vi "Main.vi"(11 "Module Admin":refnum<class "Delacor_lib_QMH_Module Admin.lvclass">) -> ()   [LabVIEW 2024, in "UI.lvlib"]
doc: "This template is based off of the Queued Message Handler design pattern and the Queued Message Handler project template that ships with LabVIEW.\n\nThe main difference is that the queue is private to this module and communication between modules is performed via Broadcast and Request events.\n\nRequest events are wrapped in public API methods and are handled in the Event Handling Loop (EHL) of this VI. Any module can register for Broadcast events sent by this module. The EHL generates messages based on user interface actions.\n\nThe Message Handling Loop (MHL) processes messages generated by the EHL, or by other messages. The messages are string values, so new messages can be added easily to the Message Cases case structure in the MHL. Each message cluster can also provide an optional value for Message Data, which is a variant that can be converted to whatever message-specific data is required.\n_____\nBased on DQMH Project Template 7.0.1.1316."
uses:
  UI.lvlib
  <vilib>/Delacor/Delacor QMH/Libraries/Message Queue_class/Delacor_lib_QMH_Message Queue.lvclass/Delacor_lib_QMH_Message Queue.ctl
  <vilib>/Delacor/Delacor QMH/Libraries/Module Admin_class/Delacor_lib_QMH_Module Admin.lvclass/Delacor_lib_QMH_Module Admin.ctl
  UI Module Template/Start Module.vi
  UI Module Template/Stop Module.vi
  <vilib>/Delacor/Delacor QMH/Libraries/Message Queue_class/Delacor_lib_QMH_Message Queue.lvclass
  Module Data--cluster.ctl
  <vilib>/Delacor/Delacor QMH/Libraries/Message Queue_class/Delacor_lib_QMH_Enqueue Message (Single).vi
  Stop Argument--cluster.ctl
  <vilib>/Delacor/Delacor QMH/Libraries/Module Admin_class/Delacor_lib_QMH_Module Admin.lvclass
  Start Modules Argument--cluster.ctl
  Modules.ctl
  Display Module Argument--cluster.ctl
  Acquire/Acquire.lvlib
  Explore/Explore.lvlib
  ListViewer/Obtain Broadcast Events for Registration.vi
  ListViewer/ListViewer.lvlib
  DataViewer/Obtain Broadcast Events for Registration.vi
  DataViewer/DataViewer.lvlib
  UI Module Template/UI Module Template.lvlib
panel:
  in  "Buttons":bool[](array[boolean])
  in  "Explore":bool
  in  "Acquisition":bool
  out "Status":string
  out "error out":errorcluster
  out "Status":string
  in  "Simulate MHL Error":bool
  in  "Simulate EHL Error":bool
  # "DQMH UI Demo"
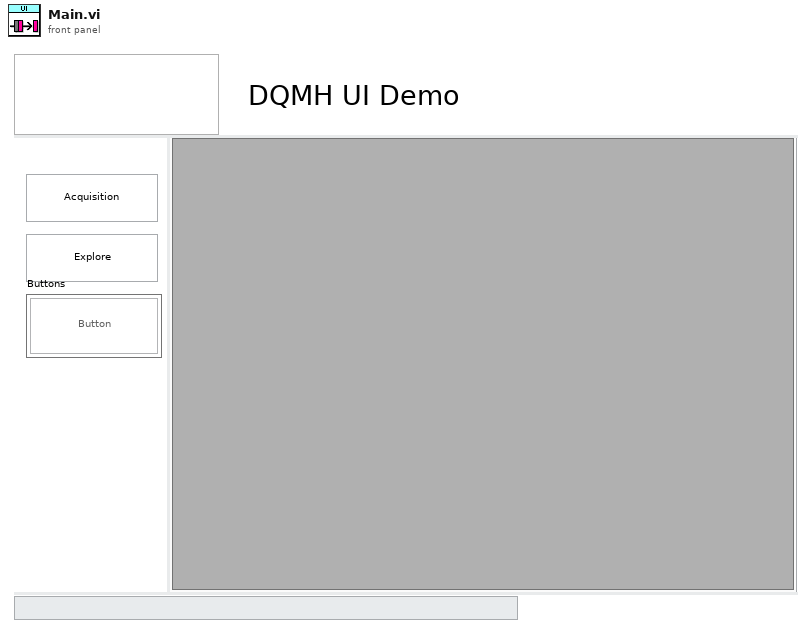
[diagram p1: front panel]
types:
  T1 = typedef "UI.lvlib/Module Data--cluster.ctl" = cluster{"Status":string, "Modules":refnum<vi>[]}
  T2 = typedef "UI.lvlib/Request Events--cluster.ctl" = cluster{"Stop Module":refnum<user-event>, "Show Panel":refnum<user-event>, "Hide Panel":refnum<user-event>, "Get Module Execution Status":refnum<user-event>, "Show Diagram":refnum<user-event>, "Private":cluster{"Start Modules":refnum<user-event>}, "Display Module":refnum<user-event>}
  T3 = typedef "ListViewer.lvlib/Broadcast Events--cluster.ctl" = cluster{"Module Did Init":refnum<user-event>, "Status Updated":refnum<user-event>, "Error Reported":refnum<user-event>, "Module Did Stop":refnum<user-event>, "Update Module Execution Status":refnum<user-event>}
  T4 = typedef "DataViewer.lvlib/Broadcast Events--cluster.ctl" = cluster{"Module Did Init":refnum<user-event>, "Status Updated":refnum<user-event>, "Error Reported":refnum<user-event>, "Module Did Stop":refnum<user-event>, "Update Module Execution Status":refnum<user-event>}
  T5 = enum32{"invalid lock state", "Not Locked", "Locked (No Password)", "Password-protected"}
  T6 = typedef "UI.lvlib/Stop Argument--cluster.ctl" = cluster{"Origin":string, "Exit via Stop Module Req?":bool, "Wait for Module to stop?":bool}
  T7 = typedef "UI.lvlib/Start Modules Argument--cluster.ctl" = cluster{"Boolean":bool}
  T8 = typedef "UI.lvlib/Display Module Argument--cluster.ctl" = cluster{"Modules":T9}
  T9 = typedef "UI.lvlib/Modules.ctl" = enum16{"Explore", "Acquisition"}
  T10 = enum32{"Invalid", "Standard", "Closed", "Hidden", "Minimized", "Maximized"}
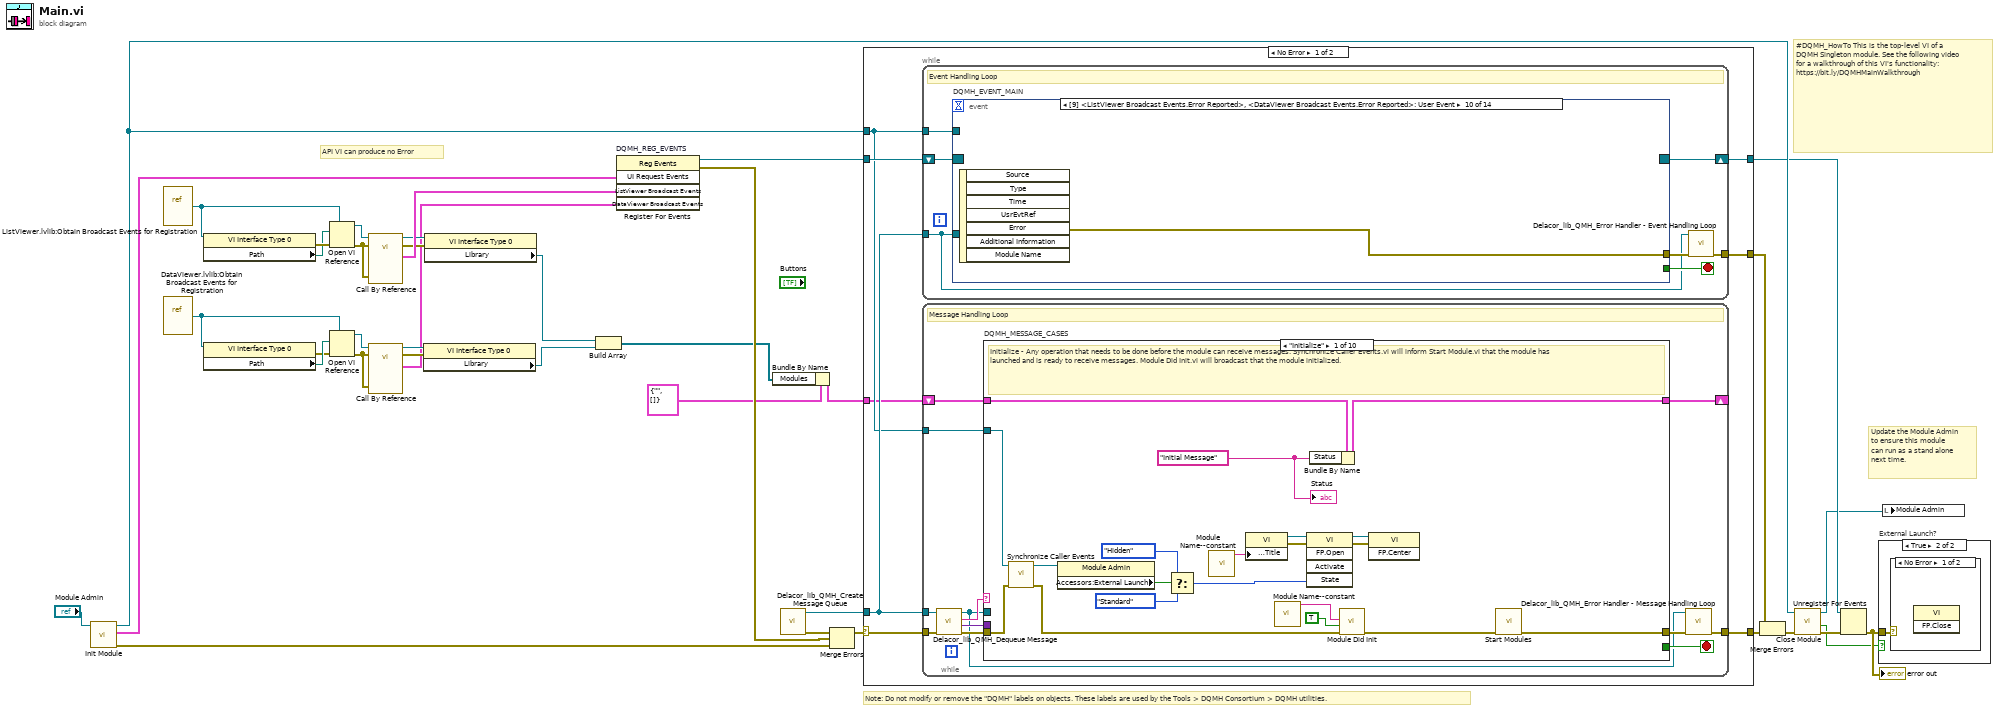
[diagram p0: block diagram]
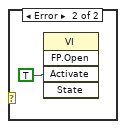
[diagram p3: hidden frame]
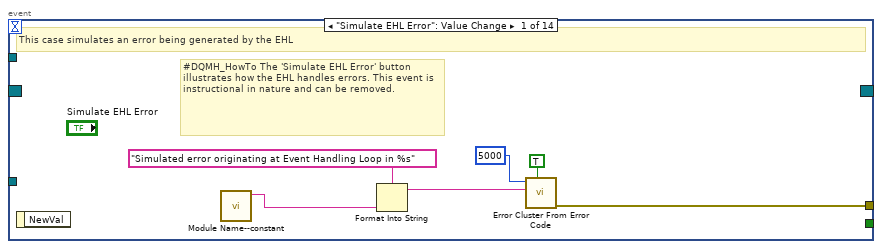
[diagram p4: hidden frame]
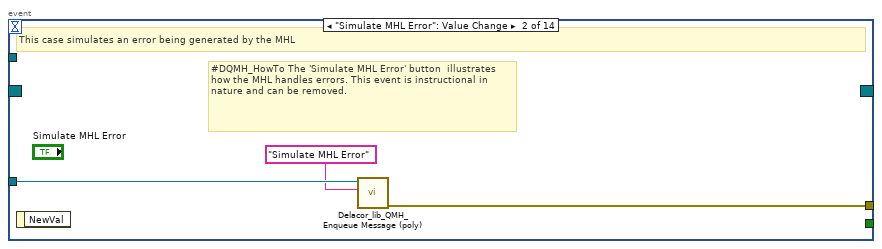
[diagram p5: hidden frame]
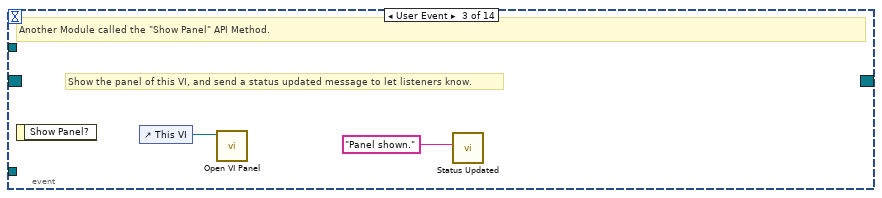
[diagram p6: hidden frame]
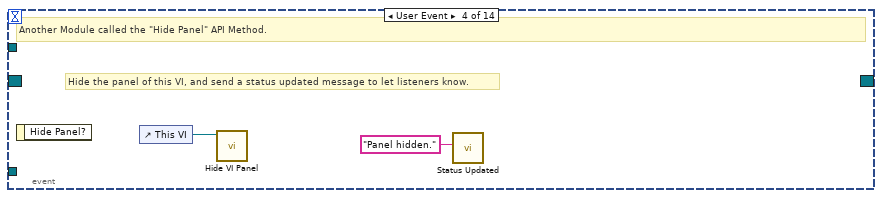
[diagram p7: hidden frame]
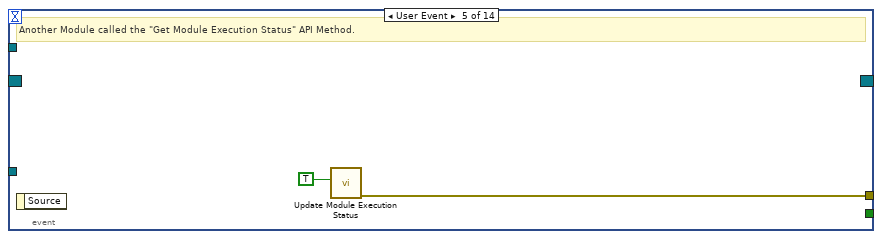
[diagram p8: hidden frame]
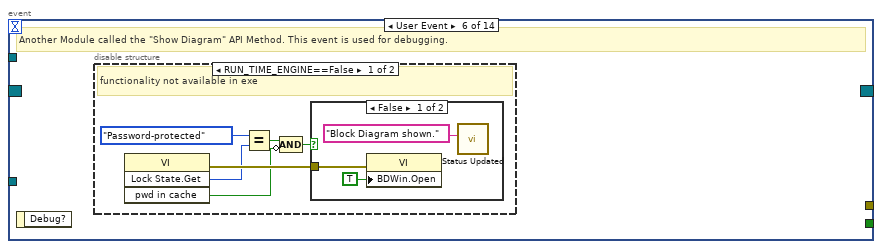
[diagram p9: hidden frame]
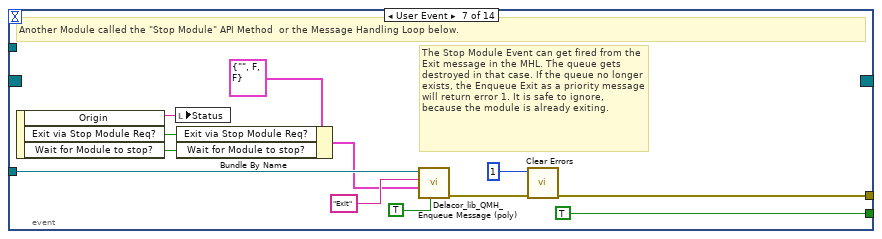
[diagram p12: hidden frame]
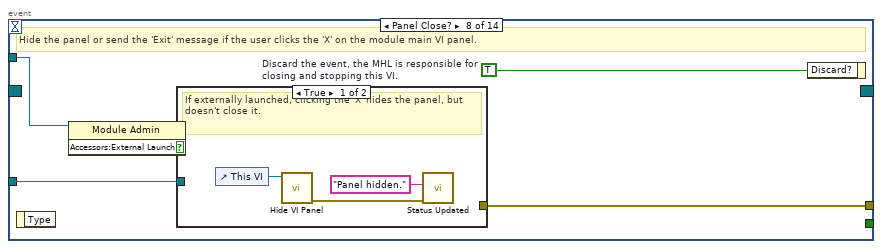
[diagram p13: hidden frame]
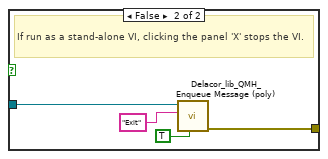
[diagram p14: hidden frame]
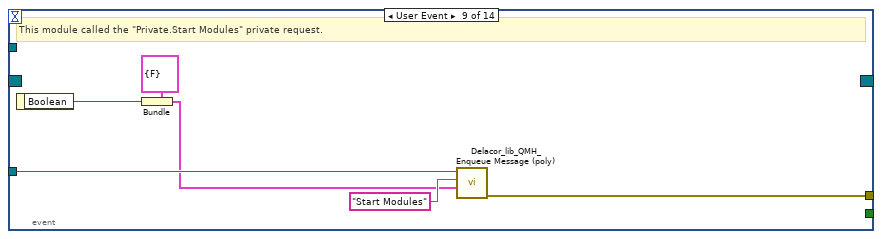
[diagram p15: hidden frame]
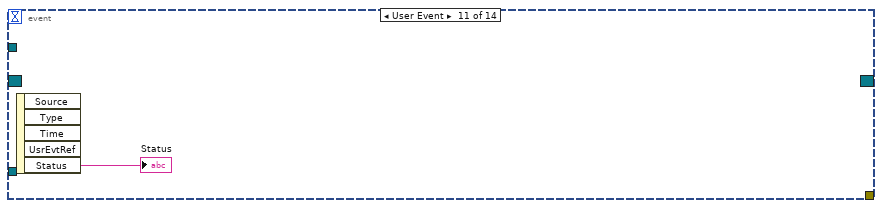
[diagram p16: hidden frame]
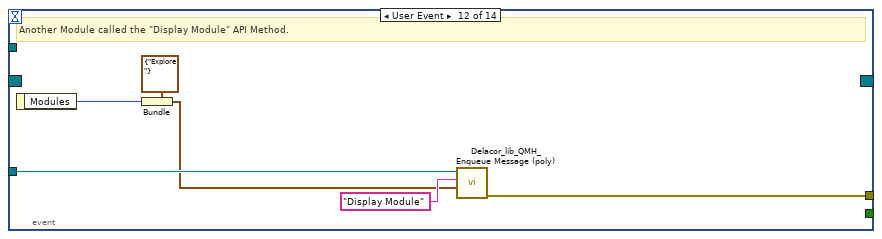
[diagram p17: hidden frame]
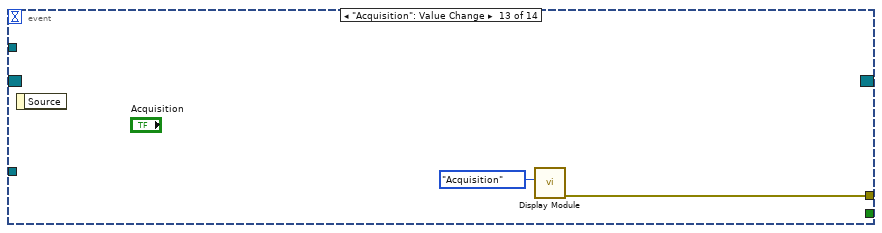
[diagram p18: hidden frame]
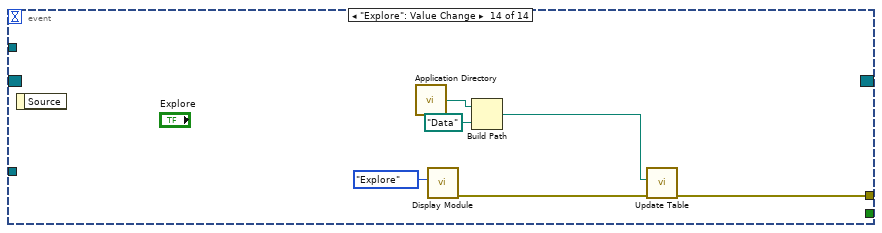
[diagram p19: hidden frame]
diagram:
  # "API VI can produce no Error"
  # "#DQMH_HowTo This is the top-level VI of a DQMH Singleton module. See the following video for a walkthrough of this VI's functionality: https://bit.ly/DQMHMainWalkthrough"
  # "Note: Do not modify or remove the \"DQMH\" labels on objects. These labels are used by the Tools > DQMH Consortium > DQMH utilities."
  # "Update the Module Admin to ensure this module can run as a stand alone next time."
  n1 = call "Init Module.vi"("Singleton Module Admin in"="Module Admin") -> ("error out"=w23:errorcluster, "UI Request Events"=w28:T2, "Singleton Module Admin out"=w31:refnum<class "Delacor_lib_QMH_Module Admin.lvclass">)  [unwired: 8 in]
  n2 = vi-ref "ListViewer.lvlib:Obtain Broadcast Events for Registration.vi"() -> (w19:refnum<vi>)
  n3 = vi-ref "DataViewer.lvlib:Obtain Broadcast Events for Registration.vi"() -> (w10:refnum<vi>)
  n4 = property class="VI Interface Type 0"(reference=w19) -> (error out=w20:errorcluster, "Path"=w18:path)  [unwired: 1 in, 1 out]
  n5 = property class="VI Interface Type 0"(reference=w10) -> (error out=w9:errorcluster, "Path"=w11:path)  [unwired: 1 in, 1 out]
  n6 = Open VI Reference(type specifier VI Refnum (for type only)=w19, vi path=w18, error in (no error)=w20) -> (vi reference=w21:refnum<vi>, error out=w16:errorcluster)  [unwired: 3 in]
  n7 = Open VI Reference(type specifier VI Refnum (for type only)=w10, vi path=w11, error in (no error)=w9) -> (vi reference=w8:refnum<vi>, error out=w12:errorcluster)  [unwired: 3 in]
  n8 = call-by-ref "?"(reference=w21, error in=w16, "error in"=w16) -> (reference out=w15:refnum<vi>, error out=w4:errorcluster, "ListViewer Broadcast Events"=w17:T3)  [unwired: 8 in, 2 out]
  n9 = call-by-ref "?"(reference=w8, error in=w12, "error in"=w12) -> (reference out=w6:refnum<vi>, error out=w5:errorcluster, "DataViewer Broadcast Events"=w1:T4)  [unwired: 8 in, 2 out]
  n10 = property class="VI Interface Type 0"(reference=w6, error in=w5) -> ("Library"=w3:refnum<vi>)  [unwired: 2 out]
  n11 = property class="VI Interface Type 0"(reference=w15, error in=w4) -> ("Library"=w7:refnum<vi>)  [unwired: 2 out]
  n12 = Build Array(w7, w3) -> (w2:refnum<vi>[])
  n13 = register-events "DQMH_REG_EVENTS"(w28, w17, w1) -> (reference out=w29:refnum<event-registration>, error out=w22:errorcluster)  [unwired: 2 in]
  n14 = Bundle By Name(cluster=T1 {"Status"="", "Modules"=[]} ("Data Cluster"), "Modules"=w2) -> (w13:T1)
  n15 = call <vilib>:"Delacor_lib_QMH_Create Message Queue.vi"() -> ("error out"=w33:errorcluster, "Message Queue"=w27:refnum<class "Delacor_lib_QMH_Message Queue.lvclass">)  [unwired: 10 in]
  n16 = Merge Errors(w33, w22, w23) -> (w32:errorcluster)
  n17 = case shown="No Error" w32 {
    selector: w32 -> [w44 w257]
    tunnel: [w46 w256] -> w38
    tunnel: [w43 w255] -> w30
    tunnel: w29 -> [w42 w255]
    tunnel: w27 -> [w41 w250]
    tunnel: [w45 _] -> w36
    tunnel: w31 -> [w40 w251]
    tunnel: w13 -> [w39 _]
    frame No Error {
      n18 = while {
        tunnel: w41 -> [w47]
        shift-right: [w50] -> w43
        shift-left: w42 -> [w51]
        tunnel: [w52] -> w45
        tunnel: w40 -> [w48]
        stop <- w49 stop-if-true
        # "Event Handling Loop"
        n19 = event "DQMH_EVENT_MAIN" shown="[9] <ListViewer Broadcast Events.Error Reported>, <DataViewer Broadcast Events.Error Reported>: User Event" {
          selector: w51 -> [_ _ _ _ _ _ _ _ _ _ _ _ _ _]
          dyn-events: [_ _ _ _ _ _ _ _ _ _ _ _ _ _] -> w50
          timeout: _ -> [_ _ _ _ _ _ _ _ _ _ _ _ _ _]
          tunnel: [_ _ _ _ _ _ TRUE ("Discard?") _ _ _ _ _ _ _] -> w49
          tunnel: w47 -> [_ w61 _ _ _ _ w85 w92 w107 _ _ w115 _ _]
          tunnel: [w59 w62 _ _ w68 _ w88 w94 w102 w108 _ w110 w116 w121] -> w53
          tunnel: w48 -> [_ _ _ _ _ _ _ w91 _ _ _ _ _ _]
          event "Simulate EHL Error": Value Change {
            # "#DQMH_HowTo The 'Simulate EHL Error' button  illustrates how the EHL handles errors. This event is instructional in nature and can be removed."
            # "This case simulates an error being generated by the EHL"
            n20 = event-data() -> ()  [unwired: 1 in, 1 out]
            n21 = call "Module Name--constant.vi"() -> ("Module Name"=w56:string)  [unwired: 11 in]
            n22 = Format Into String(format string="Simulated error originating at Event Handling Loop in %s", w56) -> (resulting string=w57:string)  [unwired: 2 in, 1 out]
            n23 = call <vilib>:"Error Cluster From Error Code.vi"("show call chain? (False)"=TRUE, "error message (\"\")"=w57, "error code (0)"=5000) -> ("error out"=w59:errorcluster)  [unwired: 6 in]
          }
          event "Simulate MHL Error": Value Change {
            # "#DQMH_HowTo The 'Simulate MHL Error' button  illustrates how the MHL handles errors. This event is instructional in nature and can be removed."
            # "This case simulates an error being generated by the MHL"
            n24 = event-data() -> ()  [unwired: 1 in, 1 out]
            n25 = call-poly <vilib>:"Delacor_lib_QMH_Enqueue Message (poly).vi"("Message"="Simulate MHL Error", "Message Queue in"=w61) -> ("error out"=w62:errorcluster)  [unwired: 8 in, 1 out]
          }
          event User Event {
            # "Show the panel of this VI, and send a status updated message to let listeners know."
            # "Another Module called the \"Show Panel\" API Method."
            n26 = event-data() -> ()  [unwired: 1 in, 1 out]
            n27 = control-ref of="This VI"() -> (w64:refnum<vi>)
            n28 = call "Open VI Panel.vi"("VI"=w64) -> ()  [unwired: 10 in, 1 out]
            n29 = call "Status Updated.vi"("Status"="Panel shown." ("format string")) -> ()  [unwired: 10 in, 1 out]
          }
          event User Event {
            # "Hide the panel of this VI, and send a status updated message to let listeners know."
            # "Another Module called the \"Hide Panel\" API Method."
            n30 = event-data() -> ()  [unwired: 1 in, 1 out]
            n31 = control-ref of="This VI"() -> (w66:refnum<vi>)
            n32 = call "Hide VI Panel.vi"("VI"=w66) -> ()  [unwired: 10 in, 1 out]
            n33 = call "Status Updated.vi"("Status"="Panel hidden." ("format string")) -> ()  [unwired: 10 in, 1 out]
          }
          event User Event {
            # "Another Module called the \"Get Module Execution Status\" API Method."
            n34 = event-data() -> ()  [unwired: 1 in, 1 out]
            n35 = call "Update Module Execution Status.vi"("Running?"=TRUE) -> ("error out"=w68:errorcluster)  [unwired: 10 in]
          }
          event User Event {
            # "Another Module called the \"Show Diagram\" API Method. This event is used for debugging."
            n36 = event-data() -> ()  [unwired: 1 in, 1 out]
            n37 = disable-structure shown="RUN_TIME_ENGINE==False" {
              frame condition #0 (active) {
                # "functionality not available in exe"
                n38 = invoke on="Invoke Node" class="VI" method="Lock State.Get"() -> (error out=w74:errorcluster, "Get Lock State"=w73:T5, "pwd in cache"=w70:bool)  [unwired: 4 in, 1 out]
                n39 = Equal?(x=T5."Password-protected", y=w73) -> (x = y?=w71:bool)
                n40 = Compound Arithmetic op=AND(w71, invert w70) -> (w69:bool)
                n41 = case shown="False" w69 {
                  tunnel: w74 -> [w77 _]
                  frame False {
                    n42 = property on="Property Node" class="VI"(error in=w77, "BDWin.Open"=TRUE ("Block Diagram Window:Open")) -> ()  [unwired: 1 in, 2 out]
                    n43 = call "Status Updated.vi"("Status"="Block Diagram shown." ("format string")) -> ()  [unwired: 10 in, 1 out]
                  }
                  frame True {
                    # "Password-protected VI, and the password is not in the cache. Do not show the diagram."
                  }
                }
              }
              frame condition #1 {
              }
            }
          }
          event User Event {
            # "The Stop Module Event can get fired from the Exit message in the MHL. The queue gets destroyed in that case. If the queue no longer exists, the Enqueue Exit as a priority message will return error 1. It is safe to ignore, because the module is already exiting."
            # "Another Module called the \"Stop Module\" API Method  or the Message Handling Loop below."
            n44 = event-data() -> ("Origin"=w84:string, "Exit via Stop Module Req?"=w80:bool, "Wait for Module to stop?"=w79:bool)  [unwired: 1 in]
            n45 = local write "Status"(w84) -> ()
            n46 = Bundle By Name(cluster=T6 {"Origin"="", "Exit via Stop Module Req?"=FALSE, "Wait for Module to stop?"=FALSE} ("Stop Argument"), "Exit via Stop Module Req?"=w80, "Wait for Module to stop?"=w79) -> (w78:T6)
            n47 = call-poly <vilib>:"Delacor_lib_QMH_Enqueue Message (poly).vi"("Priority Message? (F)"=TRUE, "Message Data"=w78, "Message"="Exit", "Message Queue in"=w85) -> ("error out"=w89:errorcluster)  [unwired: 6 in, 1 out]
            n48 = call <vilib>:"Clear Errors.vi"("error in (no error)"=w89, "specific error code to clear (0: all)"=1) -> ("error out"=w88:errorcluster)  [unwired: 4 in, 1 out]
          }
          event Panel Close? {
            w93 = TRUE  # Discard the event, the MHL is responsible for closing and stopping this VI.
            # "Hide the panel or send the 'Exit' message if the user clicks the 'X' on the module main VI panel."
            n49 = event-data() -> ()  [unwired: 1 in, 1 out]
            n50 = property on="Property Node" class="Module Admin"(reference=w91) -> ("Accessors:External Launch"=w90:bool)  [unwired: 1 in, 2 out]
            n51 = case shown="True" w90 {
              tunnel: w92 -> [_ w100]
              tunnel: [_ w101] -> w94
              frame True {
                # "If externally launched, clicking the 'X' hides the panel, but doesn't close it."
                n52 = control-ref of="This VI"() -> (w97:refnum<vi>)
                n53 = call "Hide VI Panel.vi"("VI"=w97) -> ("error out"=w95:errorcluster)  [unwired: 10 in]
                n54 = call "Status Updated.vi"("error in"=w95, "Status"="Panel hidden." ("format string")) -> ()  [unwired: 9 in, 1 out]
              }
              frame False {
                # "If run as a stand-alone VI, clicking the panel 'X' stops the VI."
                n55 = call-poly <vilib>:"Delacor_lib_QMH_Enqueue Message (poly).vi"("Priority Message? (F)"=TRUE, "Message"="Exit", "Message Queue in"=w100) -> ("error out"=w101:errorcluster)  [unwired: 7 in, 1 out]
              }
            }
            n56 = event-data ("Event Filter Node")("Discard?"=w93) -> ()  [unwired: 1 in, 1 out]
          }
          event User Event {
            # "This module called the \"Private.Start Modules\" private request."
            n57 = event-data() -> ("Boolean"=w103:bool)  [unwired: 1 in]
            n58 = Bundle(cluster=T7 {"Boolean"=FALSE} ("Start Modules Argument"), "Boolean"=w103) -> (w104:T7)
            n59 = call-poly <vilib>:"Delacor_lib_QMH_Enqueue Message (poly).vi"("Message Data"=w104, "Message"="Start Modules", "Message Queue in"=w107) -> ("error out"=w102:errorcluster)  [unwired: 7 in, 1 out]
          }
          event User Event {
            n60 = event-data() -> ("Error"=w108:errorcluster)  [unwired: 1 in, 6 out]
          }
          event User Event {
            n61 = event-data() -> ("Status"=→"Status":string)  [unwired: 1 in, 4 out]
          }
          event User Event {
            # "Another Module called the \"Display Module\" API Method."
            n62 = event-data() -> ("Modules"=w111:T9)  [unwired: 1 in]
            n63 = Bundle(cluster=T8 {"Modules"=enum."Explore"} ("Display Module Argument"), "Modules"=w111) -> (w112:T8)
            n64 = call-poly <vilib>:"Delacor_lib_QMH_Enqueue Message (poly).vi"("Message Data"=w112, "Message"="Display Module", "Message Queue in"=w115) -> ("error out"=w110:errorcluster)  [unwired: 7 in, 1 out]
          }
          event "Acquisition": Value Change {
            n65 = event-data() -> ()  [unwired: 1 in, 1 out]
            n66 = call "Display Module.vi"("Modules"=Modules."Acquisition") -> ("error out"=w116:errorcluster)  [unwired: 10 in]
          }
          event "Explore": Value Change {
            n67 = event-data() -> ()  [unwired: 1 in, 1 out]
            n68 = call <vilib>:"Application Directory.vi"() -> ("Application Directory"=w119:path)
            n69 = call "Display Module.vi"("Modules"=Modules."Explore") -> ("error out"=w122:errorcluster)  [unwired: 10 in]
            n70 = Build Path(base path=w119, name or relative path=path "Data") -> (appended path=w118:path)
            n71 = call "Update Table.vi"("error in"=w122, "Log Folder"=w118) -> ("error out"=w121:errorcluster)  [unwired: 9 in]
          }
        }
        n72 = call-dynamic "Delacor_lib_QMH_Error Handler - Event Handling Loop.vi"("error in"=w53, "Message Queue in"=w47) -> ("dup error in"=w52:errorcluster)  [unwired: 8 in, 1 out]
      }
      n73 = while {
        tunnel: w41 -> [w124]
        shift-right: [w132] -> _
        shift-left: w39 -> [w133]
        tunnel: w44 -> [w135]
        tunnel: [w127] -> w46
        tunnel: w40 -> [w128]
        stop <- w131 stop-if-true
        # "Message Handling Loop"
        n74 = call-dynamic "Delacor_lib_QMH_Dequeue Message.vi"("error in"=w135, "Message Queue in"=w124) -> ("error out"=w134:errorcluster, "Message Data"=w129:variant, "Message"=w130:string, "Message Queue out"=w125:refnum<class "Delacor_lib_QMH_Message Queue.lvclass">)  [unwired: 6 in]
        n75 = case "DQMH_MESSAGE_CASES" shown="\"Initialize\"" w130 {
          selector: w130 -> [_ _ _ _ _ _ _ _ _ w245]
          tunnel: w125 -> [_ _ _ _ _ _ _ w211 w233 _]
          tunnel: w134 -> [w153 w157 w159 w187 w196 w198 w207 w218 w239 w248]
          tunnel: [w136 w157 w158 w179 w195 w198 w206 w214 w234 w249] -> w126
          tunnel: w133 -> [w143 w156 w161 w186 w194 w197 w204 w213 w232 w246]
          tunnel: [w142 w156 w161 w186 w194 w197 w204 w213 w232 w246] -> w132
          tunnel: [_ _ _ _ _ _ _ _ w231 _] -> w131
          tunnel: w129 -> [_ _ _ w185 _ _ _ w212 w230 _]
          tunnel: w128 -> [w144 _ _ _ _ _ _ w210 w225 _]
          frame "Initialize" {
            w138 = "Initial Message" ("Initial Message")
            # "Initialize - Any operation that needs to be done before the module can receive messages. Synchronize Caller Events.vi will inform Start Module.vi that the module has launched and is ready to receive messages. Module Did Init.vi will broadcast that the module initialized."
            n76 = call "Synchronize Caller Events.vi"("error in"=w153, "Singleton Module Admin in"=w144) -> ("error out"=w152:errorcluster, "Singleton Module Admin out"=w139:refnum<class "Delacor_lib_QMH_Module Admin.lvclass">)  [unwired: 8 in]
            n77 = property on="Property Node" class="Module Admin"(reference=w139) -> ("Accessors:External Launch"=w148:bool)  [unwired: 1 in, 2 out]
            n78 = Select(t=T10."Hidden" ("State"), s=w148, f=T10."Standard" ("State")) -> (s? t:f=w145:T10)
            n79 = call "Module Name--constant.vi"() -> ("Module Name"=w151:string)  [unwired: 11 in]
            n80 = property on="Property Node" class="VI"("Front Panel.Title"=w151) -> (reference out=w150:refnum<vi>, error out=w155:errorcluster)  [unwired: 2 in]
            n81 = call "Module Name--constant.vi"() -> ("Module Name"=w140:string)  [unwired: 11 in]
            n82 = invoke on="Invoke Node" class="VI" method="FP.Open"(reference=w150, error in=w155, "State"=w145) -> (reference out=w149:refnum<vi>, error out=w154:errorcluster)  [unwired: 2 in, 3 out]
            n83 = Bundle By Name(cluster=w143, "Status"=w138) -> (w142:T1)
            n84 = call "Module Did Init.vi"("error in"=w152, "Initialized?"=TRUE, "Origin"=w140) -> ("error out"=w137:errorcluster)  [unwired: 8 in]
            n85 = invoke on="Invoke Node" class="VI" method="FP.Center"(reference=w149, error in=w154) -> ()  [unwired: 1 in, 3 out]
            n86 = call "Start Modules.vi"("error in"=w137) -> ("error out"=w136:errorcluster)  [unwired: 10 in]
            "Status" <- w138
          }
          frame "---Module Specific---" {
            # "Separator -- The following cases handle messages specific to this Module."
          }
          frame "Start Modules" {
            # "Start all Modules."
            n87 = Unbundle By Name(w161) -> ("Modules"=w160:refnum<vi>[])
            n88 = for {
              tunnel: w160 -> [w169] mode=indexing
              shift-right: [w162] -> w158
              shift-left: w159 -> [w177]
              n89 = call "Find VI.vi"("error in (no error)"=w177, "name"="Start Module.vi" ("x"), "Library in"=w169) -> ("error out"=w176:errorcluster, "VI Reference"=w173:refnum<vi>)  [unwired: 7 in]
              n90 = vi-ref "UI Module Template.lvlib:Start Module.vi"() -> (w172:refnum<vi>)
              n91 = Open VI Reference(type specifier VI Refnum (for type only)=w172, vi path=w173, error in (no error)=w176) -> (vi reference=w171:refnum<vi>, error out=w174:errorcluster)  [unwired: 3 in]
              n92 = call-by-ref "?"(reference=w171, error in=w174) -> (error out=w170:errorcluster)  [unwired: 8 in, 5 out]
              n93 = call "Find VI.vi"("error in (no error)"=w170, "name"="Stop Module.vi", "Library in"=w169) -> ("error out"=w164:errorcluster, "VI Reference"=w163:refnum<vi>)  [unwired: 7 in]
              n94 = vi-ref "UI Module Template.lvlib:Stop Module.vi"() -> (w166:refnum<vi>)
              n95 = Open VI Reference(type specifier VI Refnum (for type only)=w166, vi path=w163, error in (no error)=w164) -> (vi reference=w167:refnum<vi>, error out=w165:errorcluster)  [unwired: 3 in]
              n96 = call-by-ref "?"(reference=w167, error in=w165) -> (error out=w162:errorcluster)  [unwired: 11 in, 2 out]
            }
          }
          frame "Display Module" {
            # "Displays the specified module in the subpanel."
            n97 = Variant To Data(error in=w187, type=T8 {"Modules"=enum."Explore"} ("Display Module Argument"), Variant=w185) -> (data=w183:T8, error out=w181:errorcluster)
            n98 = Unbundle By Name(w183) -> ("Modules"=w182:T9)
            n99 = case shown="\"Explore\", Default" w182 {
              tunnel: [w190 w192] -> w180
              tunnel: [w189 w193] -> w178
              tunnel: w181 -> [w188 w191]
              frame "Explore", Default {
                n100 = call "Get Reference.vi"("error in"=w188) -> ("error out"=w190:errorcluster, "VI Refnum"=w189:refnum<vi>)  [unwired: 8 in, 1 out]
              }
              frame "Acquisition" {
                n101 = call "Get Reference.vi"("error in"=w191) -> ("error out"=w192:errorcluster, "Main VI"=w193:refnum<vi>)  [unwired: 8 in, 1 out]
              }
            }
            n102 = invoke on="Sub Panel" class="SubPnl" method="Insert VI"(error in=w180, "VI Ref"=w178) -> (error out=w179:errorcluster)  [unwired: 2 in, 3 out]
          }
          frame "---Copy This Frame---" {
            # "Duplicate this frame when creating new messages.  Change this comment in the duplicated frame to describe this message."
            n103 = Merge Errors(w196) -> (w195:errorcluster)
          }
          frame "---Exit and Error Handling---" {
            # "Separator - The following cases handle errors and exit messages."
          }
          frame "Simulate MHL Error" {
            # "#DQMH_HowTo The 'Simulate MHL Error' button  illustrates how the MHL handles errors. This event is instructional in nature and can be removed."
            # "Simulate an error occurring at the MHL"
            n104 = call "Module Name--constant.vi"() -> ("Module Name"=w200:string)  [unwired: 11 in]
            n105 = Format Into String(format string="Simulated error originating at Message Handling Loop in %s", w200) -> (resulting string=w201:string)  [unwired: 2 in, 1 out]
            n106 = call <vilib>:"Error Cluster From Error Code.vi"("show call chain? (False)"=TRUE, "error message (\"\")"=w201, "error code (0)"=5001) -> ("error out"=w205:errorcluster)  [unwired: 6 in]
            n107 = Merge Errors(w207, w205) -> (w206:errorcluster)
          }
          frame "Error" {
            # "#CodeRecommended - If the module is running in standalone mode (External Launch = FALSE), this code will pop up an error dialog and call the 'Exit' message if an error occurs. Add more fine-grained error management here."
            # "Error - Check the error message data and respond accordingly. This message is sent by the \"Error Handler\" VIs at the end of each loop in this application."
            n108 = Variant To Data(error in=w218, type=errorcluster {"status"=FALSE, "code"=0, "source"=""} ("error constant"), Variant=w212) -> (data=w208:errorcluster, error out=w216:errorcluster)
            n109 = property on="Property Node" class="Module Admin"(reference=w210) -> ("Accessors:External Launch"=w209:bool)  [unwired: 1 in, 2 out]
            n110 = local write "error out"(w208) -> ()
            n111 = call "Error Reported.vi"("Error"=w208) -> ()  [unwired: 10 in, 1 out]
            n112 = case shown="False" w209 {
              tunnel: [w223 _] -> w215
              tunnel: w211 -> [w221 _]
              tunnel: w208 -> [w222 _]
              frame False {
                n113 = disable-structure shown="Default" {
                  disable-tunnel: w222 -> [w224 _]
                  frame condition #0 (active) {
                    # "If the module is running standalone, then pop up an error dialog and call the \"Exit\" message."
                    n114 = call <vilib>:"Simple Error Handler.vi"("error in (no error)"=w224) -> ()  [unwired: 4 in, 5 out]
                  }
                  frame condition #1 {
                    # "To prevent the Simple Error Handler VI from being loaded (e.g. when deploying to a Real-Time target), add the Conditional Disable Symbol \"DQMH_Disable_SEH\" to your project and set it to TRUE."
                  }
                }
                n115 = call-poly <vilib>:"Delacor_lib_QMH_Enqueue Message (poly).vi"("Priority Message? (F)"=TRUE, "Message"="Exit", "Message Queue in"=w221) -> ("error out"=w223:errorcluster)  [unwired: 7 in, 1 out]
              }
              frame True {
                # "If the module was launched externally, calling the Error Reported broadcast VI is the only action performed by the \"Error\" message. The module's caller can then process the error appropriately."
              }
            }
            n116 = Merge Errors(w216, w215) -> (w214:errorcluster)
          }
          frame "Exit" {
            w229 = 91  # 91: not all Exit messages will have an argument
            w231 = TRUE  # Stop the VI
            # "Release the message queue reference"
            # "Exit - Exit the application."
            n117 = Variant To Data(error in=w239, type=T6 {"Origin"="", "Exit via Stop Module Req?"=FALSE, "Wait for Module to stop?"=FALSE} ("Stop Argument"), Variant=w230) -> (data=w227:T6, error out=w236:errorcluster)
            n118 = call <vilib>:"Clear Errors.vi"("error in (no error)"=w236, "specific error code to clear (0: all)"=w229) -> ("error out"=w238:errorcluster)  [unwired: 4 in, 1 out]
            n119 = control-ref of="This VI"() -> (w226:refnum<vi>)
            n120 = call-dynamic "Delacor_lib_QMH_Release Message Queue.vi"("error in"=w238, "Message Queue"=w233) -> ("error out"=w237:errorcluster)  [unwired: 9 in]
            n121 = call "Handle Exit.vi"("Stop Argument"=w227, "Admin in"=w225, "VI reference"=w226) -> ("error out"=w235:errorcluster)  [unwired: 7 in, 1 out]
            n122 = Merge Errors(w237, w235) -> (w234:errorcluster)
            n123 = call "Error Reported.vi"("Error"=w234) -> ()  [unwired: 10 in, 1 out]
          }
          frame Default {
            # "'Default' case only runs if there is a message that isn't defined in any of the other cases.  Output a programming error."
            n124 = call "Module Name--constant.vi"() -> ("Module Name"=w244:string)  [unwired: 11 in]
            n125 = Format Into String(format string="The invalid message string \"%s\" was received in the Message Handling Loop for module \"%s\".", w245, w244) -> (resulting string=w240:string)  [unwired: 2 in, 1 out]
            n126 = call <vilib>:"Error Cluster From Error Code.vi"("show call chain? (False)"=TRUE, "error message (\"\")"=w240, "error code (0)"=1) -> ("error out"=w247:errorcluster)  [unwired: 6 in]
            n127 = Merge Errors(w248, w247) -> (w249:errorcluster)
          }
        }
        n128 = call-dynamic "Delacor_lib_QMH_Error Handler - Message Handling Loop.vi"("error in"=w126, "Message Queue in"=w125) -> ("dup error in"=w127:errorcluster)  [unwired: 8 in, 1 out]
      }
    }
    frame Error {
      # "Synchronize Caller Events.vi will inform Start Module.vi that the module has launched and will let the code calling Start Module.vi register for broadcasts and would permit the caller receive the broadcast that an error occurred at launch time."
      n129 = call-dynamic "Delacor_lib_QMH_Release Message Queue.vi"("error in"=w257, "Message Queue"=w250) -> ("error out"=w256:errorcluster)  [unwired: 9 in]
      n130 = call "Synchronize Caller Events.vi"("Singleton Module Admin in"=w251) -> ("error out"=w258:errorcluster)  [unwired: 9 in, 1 out]
      n131 = call "Module Name--constant.vi"() -> ("Module Name"=w254:string)  [unwired: 11 in]
      n132 = Format Into String(format string="An error occurred during initialization. %s is no longer running.", w254) -> (resulting string=w252:string)  [unwired: 2 in, 1 out]
      n133 = Merge Errors(w256, w258) -> (w259:errorcluster)
      n134 = call "Error Reported.vi"("Additional Information"=w252, "Error"=w259) -> ()  [unwired: 9 in, 1 out]
    }
  }
  n135 = Merge Errors(w36, w38) -> (w35:errorcluster)
  n136 = call "Close Module.vi"("error in"=w35, "Module Admin in"=w31) -> ("error out"=w37:errorcluster, "External Launch"=w24:bool, "Module Admin out"=w25:refnum<class "Delacor_lib_QMH_Module Admin.lvclass">)  [unwired: 7 in]
  n137 = Unregister For Events(event registration refnum=w30, error in=w37) -> (error out=w34:errorcluster)
  "error out" <- w34
  n138 = case "External Launch?" shown="True" w24 {
    tunnel: w34 -> [_ w260]
    frame False {
    }
    frame True {
      n139 = case shown="No Error" w260 {
        frame No Error {
          n140 = invoke on="Invoke Node" class="VI" method="FP.Close"() -> ()  [unwired: 3 in, 3 out]
        }
        frame Error {
          n141 = invoke on="Invoke Node" class="VI" method="FP.Open"("Activate"=TRUE ("Activate?")) -> ()  [unwired: 4 in, 5 out]
        }
      }
    }
  }
  n142 = local write "Module Admin"(w25) -> ()
